vi "Connection Status Global.vi"(8 "Operation":T1, 10 "Status In":bool) -> (0 "Notifier":refnum<notifier>, 2 "Connection Status":bool)   [LabVIEW 2015]
uses:
  Connection Status Global Action.ctl
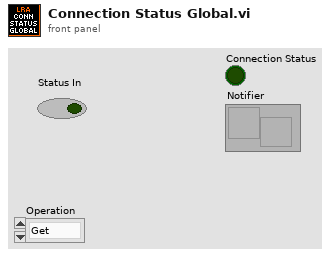
[diagram p1: front panel]
types:
  T1 = typedef "Connection Status Global Action.ctl" = enum16{"Get", "Set", "Initialize"}
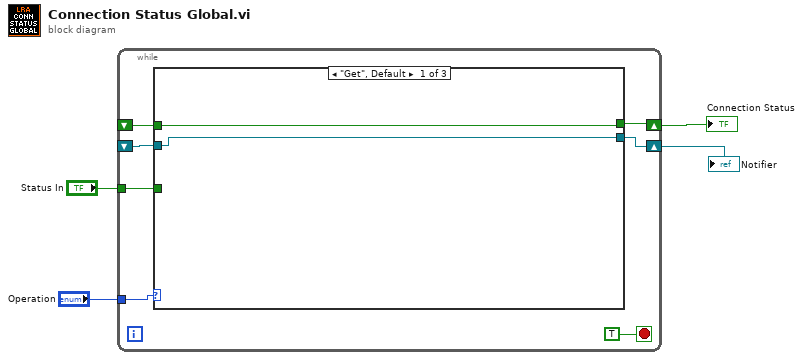
[diagram p0: block diagram]
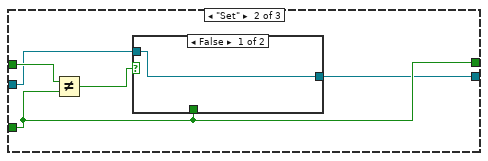
[diagram p2: hidden frame]
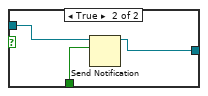
[diagram p3: hidden frame]
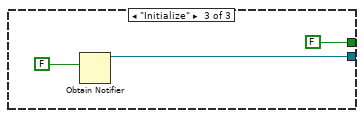
[diagram p4: hidden frame]
diagram:
  n1 = while {
    tunnel: "Operation" -> [w10]
    shift-right: [w9] -> w3
    shift-left: _ -> [w7]
    shift-right: [w8] -> w2
    shift-left: _ -> [w5]
    tunnel: "Status In" -> [w6]
    stop <- TRUE stop-if-true
    n2 = case shown="\"Get\", Default" w10 {
      tunnel: [w13 w15 FALSE] -> w9
      tunnel: [w12 w14 w23] -> w8
      tunnel: w7 -> [w13 w18 _]
      tunnel: w6 -> [_ w15 _]
      tunnel: w5 -> [w12 w16 _]
      frame "Get", Default {
      }
      frame "Set" {
        n3 = Not Equal?(x=w18, y=w15) -> (x != y?=w17:bool)
        n4 = case shown="False" w17 {
          tunnel: w16 -> [w19 w22]
          tunnel: w15 -> [_ w21]
          tunnel: [w19 w20] -> w14
          frame False {
          }
          frame True {
            n5 = Send Notification(notification=w21, notifier=w22) -> (notifier out=w20:refnum<notifier>)  [unwired: 1 in, 1 out]
          }
        }
      }
      frame "Initialize" {
        n6 = Obtain Notifier(notification data type=FALSE) -> (notifier out=w23:refnum<notifier>)  [unwired: 3 in, 2 out]
      }
    }
  }
  "Connection Status" <- w3
  "Notifier" <- w2
